vi "sub_updatePuzzle.vi"(8 "error in (no error)":errorcluster, 10 "solver array":cluster{"solved":bool, "values":string[]}[][](array[cluster]), 11 "puzzle (in)":string[][](array[string])) -> (0 "error out":errorcluster, 2 "solved ?":bool, 3 "puzzle (out)":string[][](array[string]))   [LabVIEW 2018]
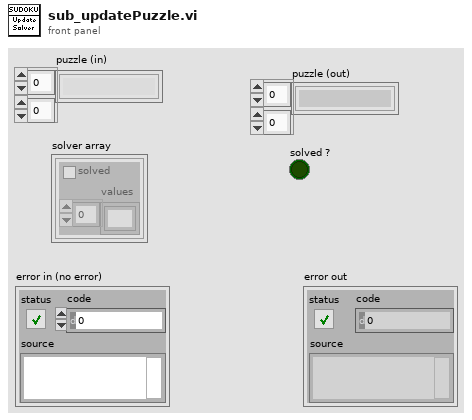
[diagram p1: front panel]
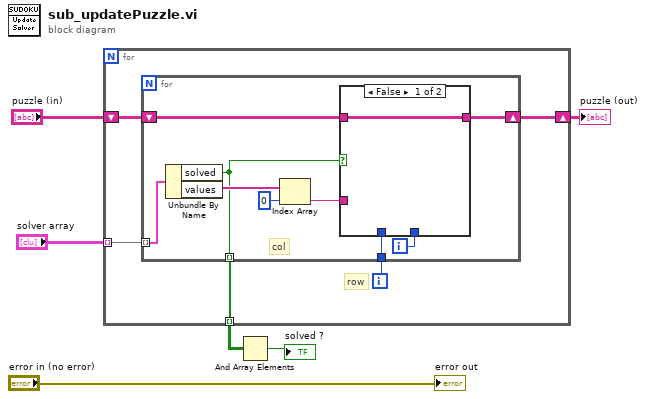
[diagram p0: block diagram]
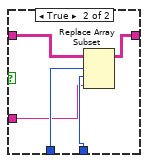
[diagram p2: hidden frame]
diagram:
  n1 = for {
    tunnel: "solver array" -> [w10] mode=indexing
    shift-right: [w8] -> w1
    shift-left: "puzzle (in)" -> [w11]
    tunnel: [w7] -> w3 mode=indexing
    i -> [w9]
    # "row"
    n2 = for {
      tunnel: w10 -> [w20] mode=indexing
      shift-right: [w13] -> w8
      shift-left: w11 -> [w17]
      tunnel: w9 -> [w16]
      tunnel: [w12] -> w7 mode=indexing
      i -> [w15]
      # "col"
      n3 = Unbundle By Name(w20) -> ("solved"=w12:bool, "values"=w19:string[])
      n4 = Index Array(array=w19, index=0) -> (element=w14:string)
      n5 = case shown="False" w12 {
        tunnel: w17 -> [w21 w26]
        tunnel: w16 -> [_ w25]
        tunnel: w15 -> [_ w24]
        tunnel: w14 -> [_ w23]
        tunnel: [w21 w22] -> w13
        frame False {
        }
        frame True {
          n6 = Replace Array Subset(array=w26, new element=w23, index (row)=w25, index (col)=w24) -> (w22:string[][])
        }
      }
    }
  }
  "puzzle (out)" <- w1
  n7 = And Array Elements(Boolean array=w3) -> (logical AND=→"solved ?":bool)
  "error out" <- "error in (no error)"
